vi "Sub Super Duper_12_09_10a_JW.vi"(0 "VISA resource name":refnum<visa-resource-name>="GPIB0::17::INSTR", 1 "Sample Properties:":T7 {"Date Created" format="%<%Y/%m/%d>T"}, 2 "TRF Cluster":T8={"Step 4"=-38.0, "# of Loops"=1.0, "Transfer 2"=FALSE, "Start 4"=-2.0, "Total Points 2"=2, "Start 3"=40.0, "Stop 2"=-40.0, "Step 3"=-1.0, "Loop Step"=0.0, "Integration Time 3"=0, "Loop Wait"=0.0, "First Step"=0.0} {"Loop Wait" format="%<%H:%M:%S>t"; "Integration Time 3" scale=0.0..2.0; "Step 3" format="%.2f"; "Stop 2" format="%.2f"; "Start 3" format="%.2f"; "Start 4" format="%.2f"; "Step 4" format="%.2f"}, 3 "TSP Cluster":T9={"Transport"=FALSE, "Start 2"=0.0, "Stop 3"=-60.0, "Step 2"=-1.0, "Start"=0.0, "Step"=-10.0, "Total Points"=7, "Integration Time"=0} {"Integration Time" scale=0.0..2.0; "Step" format="%.2f"; "Start" format="%.2f"; "Step 2" format="%.2f"; "Stop 3" format="%.2f"; "Start 2" format="%.2f"}, 4 "Compliance Cluster":T4={"Var1 sweep settings"={"sweep spacing (linear: 0)"=0, "sweep mode"=FALSE, "compliance (V)"=100.0, "compliance (A)"=0.001}, "Var1 sweep settings 2"={"sweep spacing (linear: 0)"=0, "sweep mode"=FALSE, "compliance (V)"=100.0, "compliance (A)"=0.001}, "Var2 step settings 2"={"compliance (A)"=0.001, "compliance (V)"=100.0}, "Var2 step settings"={"compliance (A)"=0.001, "compliance (V)"=100.0}} {"Var2 step settings"."compliance (V)" format="%.2f"; "Var2 step settings"."compliance (A)" format="%^.2e"; "Var2 step settings 2"."compliance (V)" format="%.2f"; "Var2 step settings 2"."compliance (A)" format="%^.2e"; "Var1 sweep settings 2"."compliance (A)" format="%^.2e"; "Var1 sweep settings 2"."compliance (V)" format="%.2f"; "Var1 sweep settings 2"."sweep spacing (linear: 0)" items=["linear", "log 10", "log 25", "log 50"]; "Var1 sweep settings"."compliance (A)" format="%^.2e"; "Var1 sweep settings"."compliance (V)" format="%.2f"; "Var1 sweep settings"."sweep spacing (linear: 0)" items=["linear", "log 10", "log 25", "log 50"]}, 5 "error in":errorcluster, 6 "Saved Folder:":path=path "C:/1DATA/2011", 7 "Wait Cluster":T3 {"Wait Time (s)" format="%.1g"; "Wait Countdown" format="%<%H:%M:%S%1u>t"}, 9 "Stop \nCountdown":bool, 11 "Loop Count":dbl, 12 "Gate Current Cluster":T1={"Gate Current (TSP)"={"Y2 axis on/off"=FALSE, "MINIMUM"=0.0, "MAXIMUM"=1.0, "Variable name"="Ig", "LIN or LOG axis"="LIN"}, "Gate Current (TRF)"={"Y2 axis on/off"=FALSE, "MINIMUM"=0.0, "MAXIMUM"=1.0, "Variable name"="Ig", "LIN or LOG axis"="LIN"}} {"Gate Current (TSP)"."MAXIMUM" format="%.9f"; "Gate Current (TSP)"."MINIMUM" format="%.9f"; "Gate Current (TRF)"."MAXIMUM" format="%.9f"; "Gate Current (TRF)"."MINIMUM" format="%.9f"}, 13 "Dielectric Constant":dbl) -> (8 "Status Indicator":bool, 10 "Vt Cluster":T2 {"Id Max" format="%.3g"; "Vt Max" format="%.3g"; "Vt Min" format="%.3g"; "Vt Ratio" format="%.3g"}, 14 "VISA resource name out":refnum<visa-resource-name>, 15 "TRF Path":path, 16 "TSP Path":path, 17 "Graph Cluster":T5, 18 "Char Cluster":T6 {"Mobility-Lin" format="%#_4e"; "On/Off" format="%#_4e"; "Mobility-Sat" format="%#_4e"}, 19 "error out":errorcluster)   [LabVIEW 2012]
uses:
  <vilib>/Platform/TimedLoop/XDataNode/wakeup.ctl
  <vilib>/Platform/TimedLoop/XDataNode/XDNodeRunTimeDep.lvlib
  <vilib>/Platform/TimedLoop/XDataNode/nitl_modes.ctl
  <vilib>/Platform/TimedLoop/XDataNode/timing_clust.ctl
  <vilib>/Platform/TimedLoop/XDataNode/XDataNode.xnode
panel:
  out "LKG Path":path
  # "Vg Sweep"
  # "Vd Step"
  # "Loops and Integration Time"
  # "Device Characteristics"
  # "Sample Properties:"
  # "%"
  # "nm"
  # "Device Properties:"
  # "um"
  # "um"
  # "Vg Step"
  # "Vd Step"
  # "Integration Time"
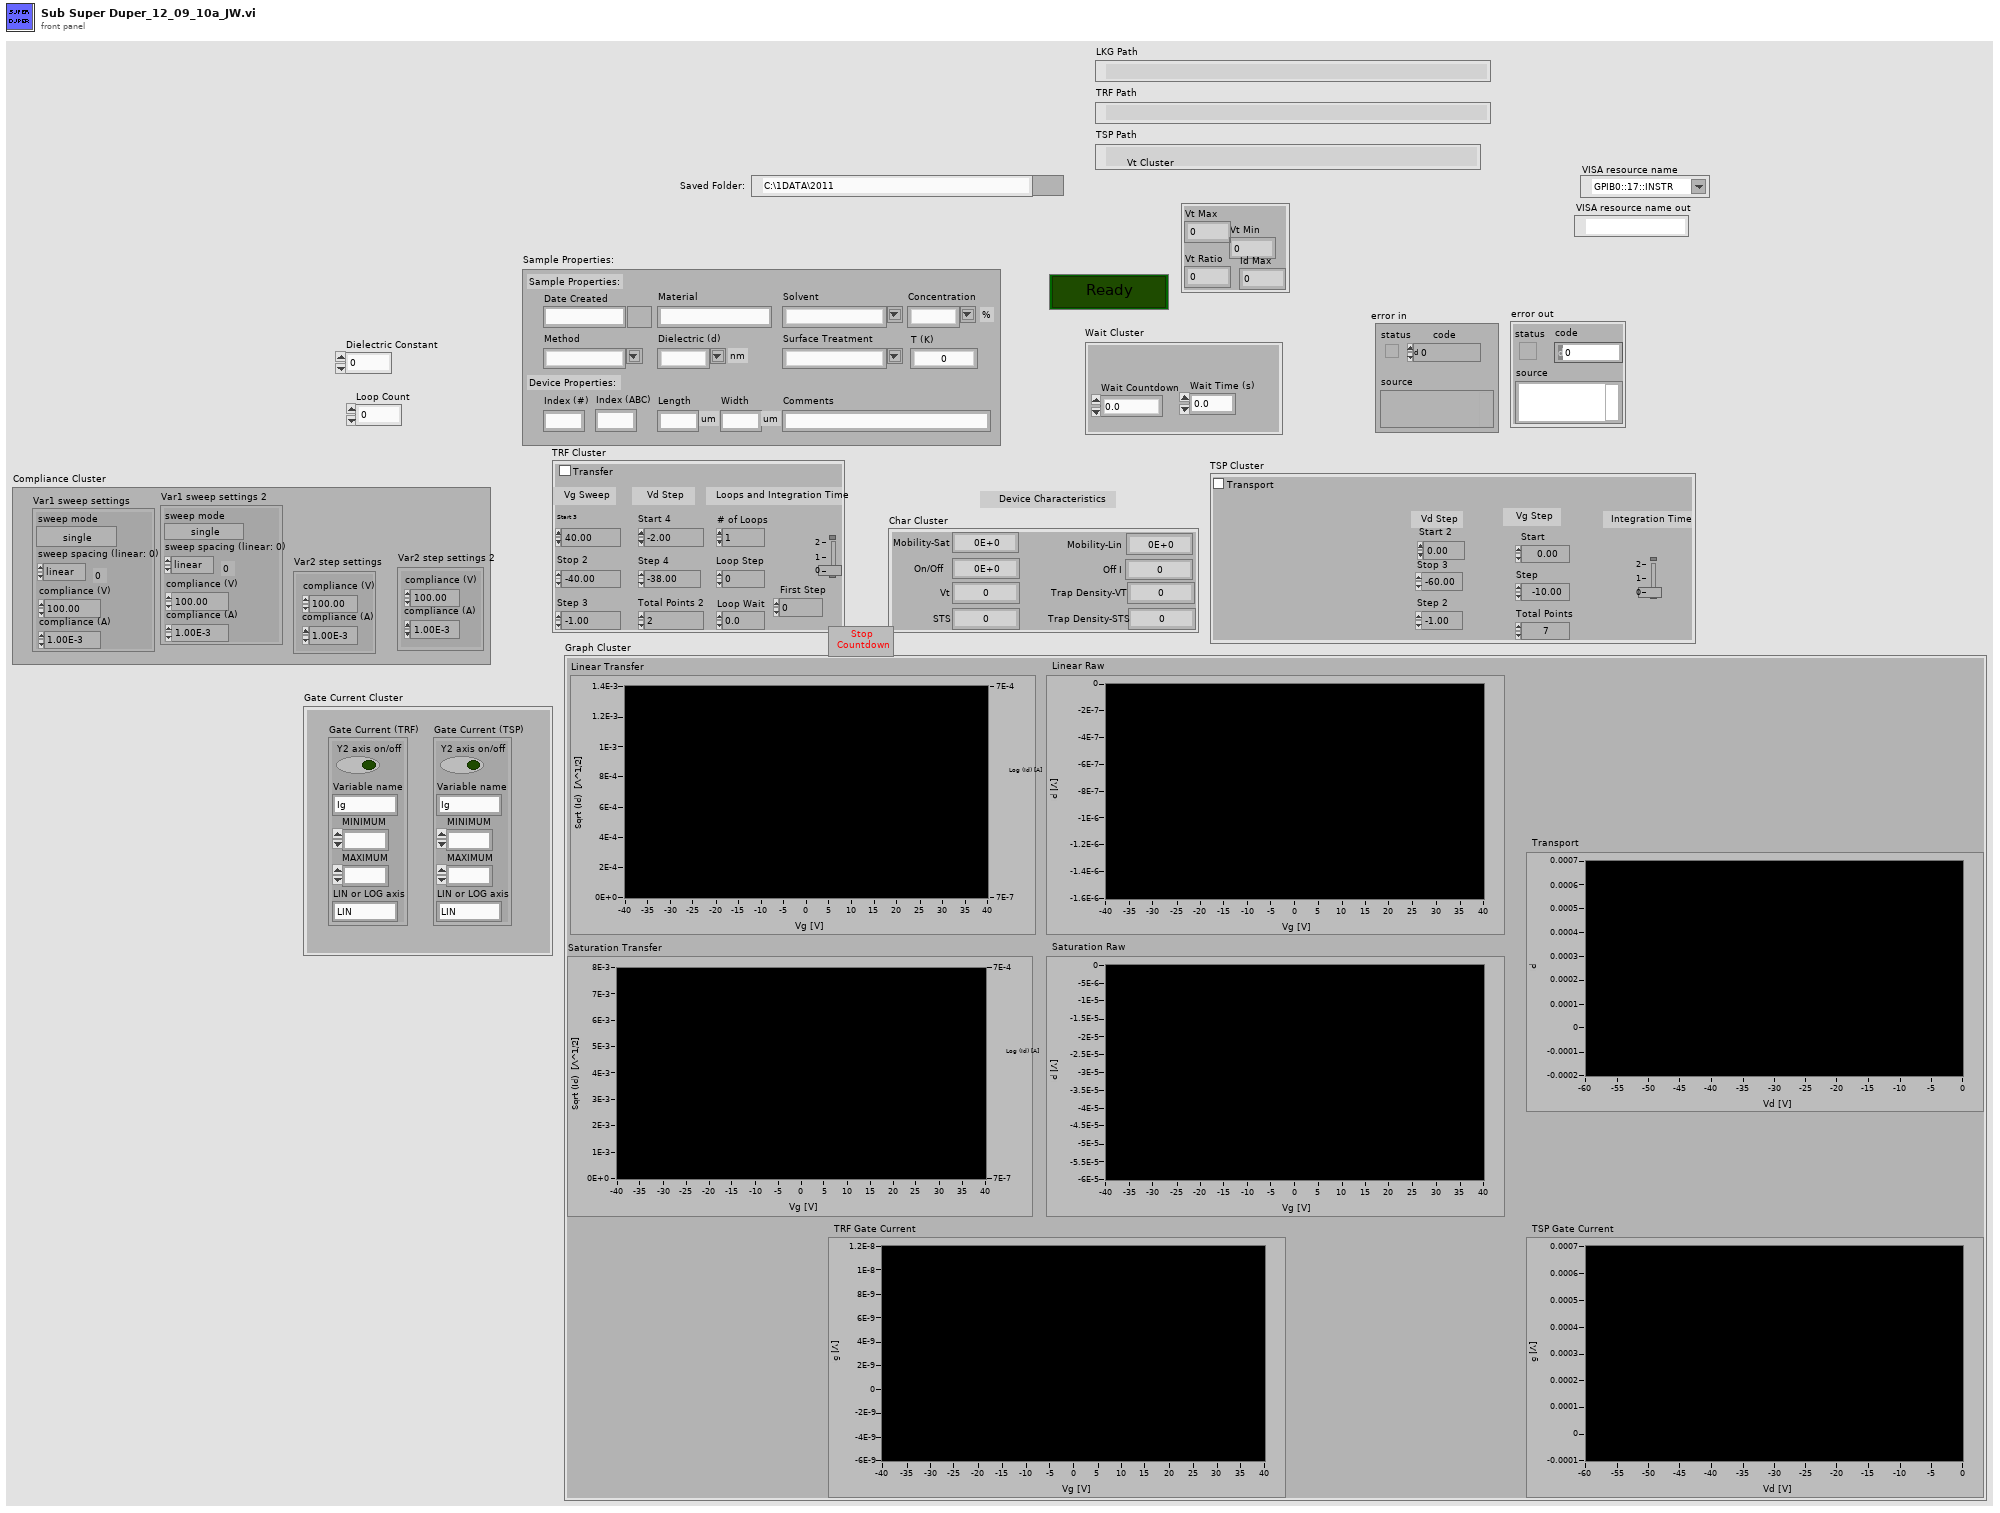
[diagram p1: front panel]
types:
  T1 = cluster{"Gate Current (TSP)":cluster{"Y2 axis on/off":bool, "MINIMUM":ext, "MAXIMUM":ext, "Variable name":string, "LIN or LOG axis":string}, "Gate Current (TRF)":cluster{"Y2 axis on/off":bool, "MINIMUM":ext, "MAXIMUM":ext, "Variable name":string, "LIN or LOG axis":string}}
  T2 = cluster{"Vt Max":i32, "Vt Min":i32, "Vt Ratio":i32, "Id Max":i32}
  T3 = cluster{"Wait Countdown":dbl, "Wait Time (s)":dbl}
  T4 = cluster{"Var1 sweep settings":cluster{"sweep spacing (linear: 0)":u16, "sweep mode":bool, "compliance (V)":dbl, "compliance (A)":dbl}, "Var1 sweep settings 2":cluster{"sweep spacing (linear: 0)":u16, "sweep mode":bool, "compliance (V)":dbl, "compliance (A)":dbl}, "Var2 step settings 2":cluster{"compliance (A)":dbl, "compliance (V)":dbl}, "Var2 step settings":cluster{"compliance (A)":dbl, "compliance (V)":dbl}}
  T5 = cluster{"Linear Transfer":cluster{dbl[], "trace":dbl[]}[], "Linear Raw":cluster{dbl[], dbl[]}[], "Saturation Transfer":cluster{dbl[], "trace":dbl[]}[], "Saturation Raw":cluster{dbl[], dbl[]}[], "Transport":cluster{dbl[], dbl[]}[], "TRF Gate Current":cluster{dbl[], dbl[]}[], "TSP Gate Current":cluster{dbl[], dbl[]}[]}
  T6 = cluster{"Mobility-Sat":dbl, "Mobility-Lin":dbl, "On/Off ":dbl, "Off I":dbl, "Vt":dbl, "STS":dbl, "Trap Density-VT":dbl, "Trap Density-STS":dbl}
  T7 = cluster{"Date Created":timestamp, "Material":string, "Solvent":string, "Concentration":string, "Method":string, "Dielectric (d)":string, "Index (#)":string, "Index (ABC)":string, "Length":string, "Width":string, "Surface Treatment":string, "Comments":string, "T (K)":dbl}
  T8 = cluster{"Step 4":dbl, "# of Loops":dbl, "Transfer 2":bool, "Start 4":dbl, "Total Points 2":u16, "Start 3":dbl, "Stop 2":dbl, "Step 3":dbl, "Loop Step":dbl, "Integration Time 3":u32, "Loop Wait":dbl, "First Step":dbl}
  T9 = cluster{"Transport":bool, "Start 2":dbl, "Stop 3":dbl, "Step 2":dbl, "Start":dbl, "Step":dbl, "Total Points":u16, "Integration Time":u32}
  T10 = typedef "XDNodeRunTimeDep.lvlib/timing_clust.ctl" = cluster{"Expected End [f-1]":u64, "Actual End [f-1]":u64, "Finished Late? [f-1]":bool, "Expected End [i-1]":u64, "Actual End [i-1]":u64, "Finished Late? [i-1]":bool, "Expected Start [i]":u64, "Actual Start [i]":u64, "Expected Start [f]":u64, "Actual Start [f]":u64, "Source Name":string, "Structure Name":string, "Period":i64, "Deadline":i64, "Offset":i64, "Start":i64, "Priority":i32, "Timeout":i32, "Mode":T11, "Wakeup Reason":T12, "Error":errorcluster, "Source Type":string, "Secondary Source Type":string, "Global End Time":u64, "Global Start Time":u64, "Frame Duration":u64, "Iteration Duration":u64, "Assigned CPU":i32, "I/O Scan Engine Mode":u32}
  T11 = typedef "XDNodeRunTimeDep.lvlib/nitl_modes.ctl" = enum32{"No Change", "Process missed periods, maintain original phase", "Discard missed periods, maintain original phase", "Process missed periods, ignore original phase", "Discard missed periods, ignore original phase"}
  T12 = typedef "XDNodeRunTimeDep.lvlib/wakeup.ctl" = enum32{"Normal", "Aborted", "Asynchronous wakeup", "Timing source error", "Timed loop error", "Timeout"}
  T13 = cluster{"sweep spacing (linear: 0)":u16, "sweep mode":bool, "compliance (V)":dbl, "compliance (A)":dbl}
  T14 = cluster{"compliance (A)":dbl, "compliance (V)":dbl}
  T15 = cluster{"Y2 axis on/off":bool, "MINIMUM":ext, "MAXIMUM":ext, "Variable name":string, "LIN or LOG axis":string}
  T16 = cluster{"Start 3":dbl, "Stop 2":dbl, "Step 3":dbl, "sweep spacing (linear: 0)":u16, "sweep mode":bool, "compliance (V)":dbl, "compliance (A)":dbl}
  T17 = cluster{"compliance (A)":dbl, "compliance (V)":dbl, "Start 4":dbl, "Total Points 2":u16, dbl}
  T18 = cluster{"Vt Max":i32, "Vt Min":i32, "Vt Ratio":i32, "Id Max":dbl}
  T19 = cluster{"Mobility-Sat":dbl, "Mobility-Lin":dbl, "On/Off Current":dbl, "Off I":dbl, "Vt":dbl, "STS":dbl, "Trap Density-VT":dbl, "Trap Density-STS":dbl}
  T20 = cluster{"Linear Sqrt":cluster{dbl[], "trace":dbl[]}[], "Linear Log":cluster{dbl[], "trace":dbl[]}[], "Linear Raw":cluster{dbl[], dbl[]}[], "Saturation Sqrt":cluster{dbl[], "trace":dbl[]}[], "Saturation Log":cluster{dbl[], "trace":dbl[]}[], "Saturation Raw":cluster{dbl[], "trace":dbl[]}[], "Gate Current":cluster{dbl[], "trace":dbl[]}[]}
  T21 = cluster{"Start 2":dbl, "Stop 3":dbl, "Step 2":dbl, "sweep spacing (linear: 0)":u16, "sweep mode":bool, "compliance (V)":dbl, "compliance (A)":dbl}
  T22 = cluster{"compliance (A)":dbl, "compliance (V)":dbl, "Start":dbl, "Total Points":u16, "Step":dbl}
  T23 = cluster{"Transport":cluster{dbl[], dbl[]}[], "Gate Current":cluster{dbl[], dbl[]}[]}
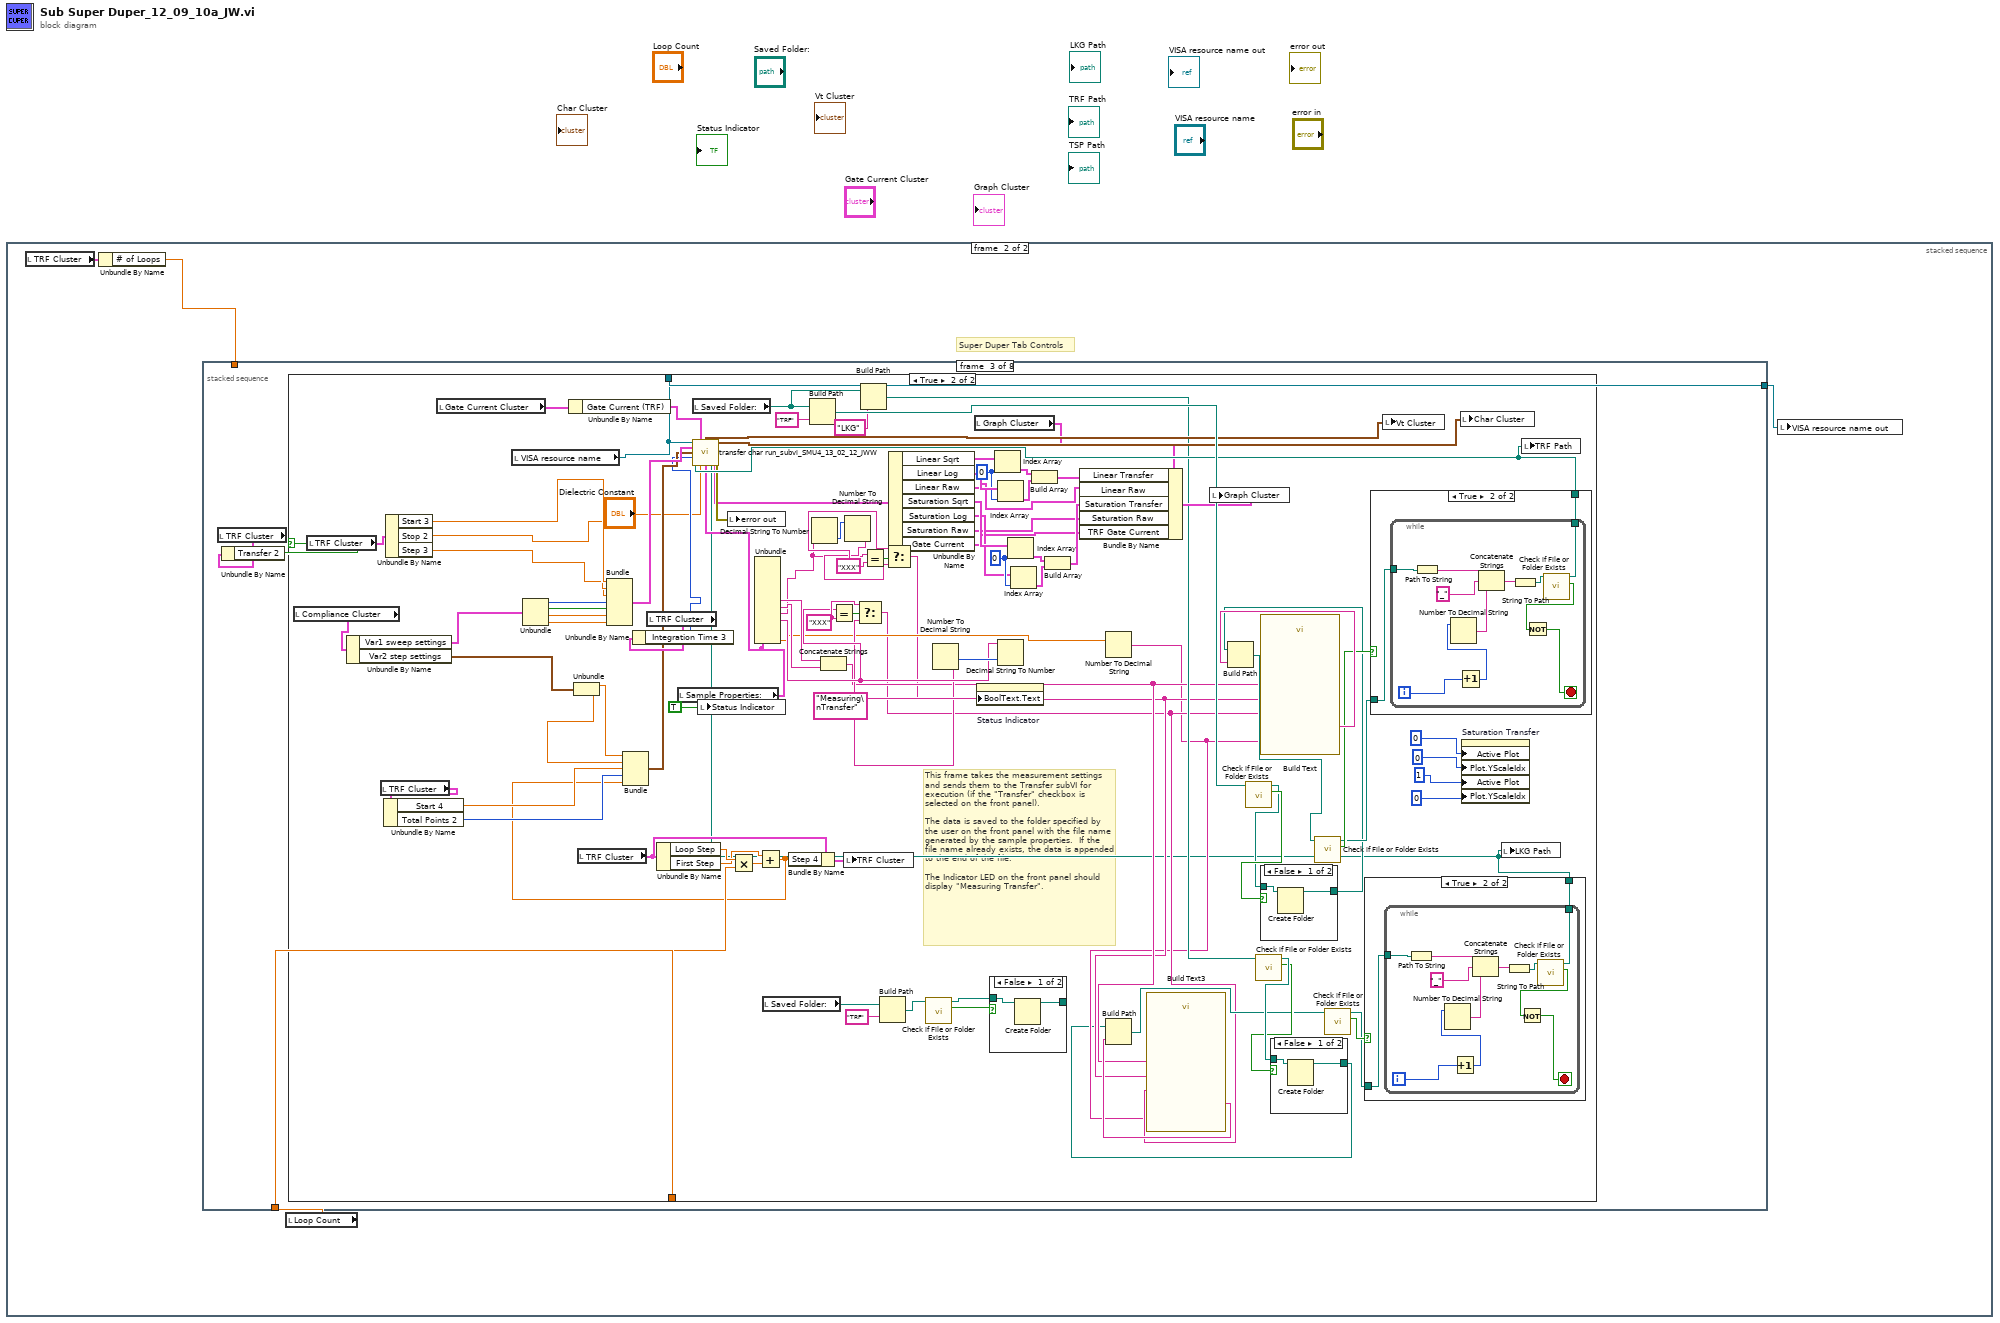
[diagram p0: block diagram]
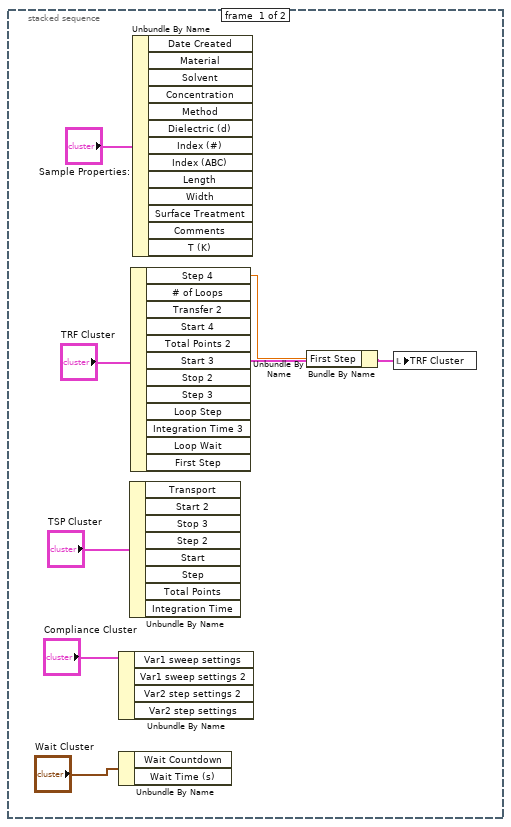
[diagram p2: hidden frame]
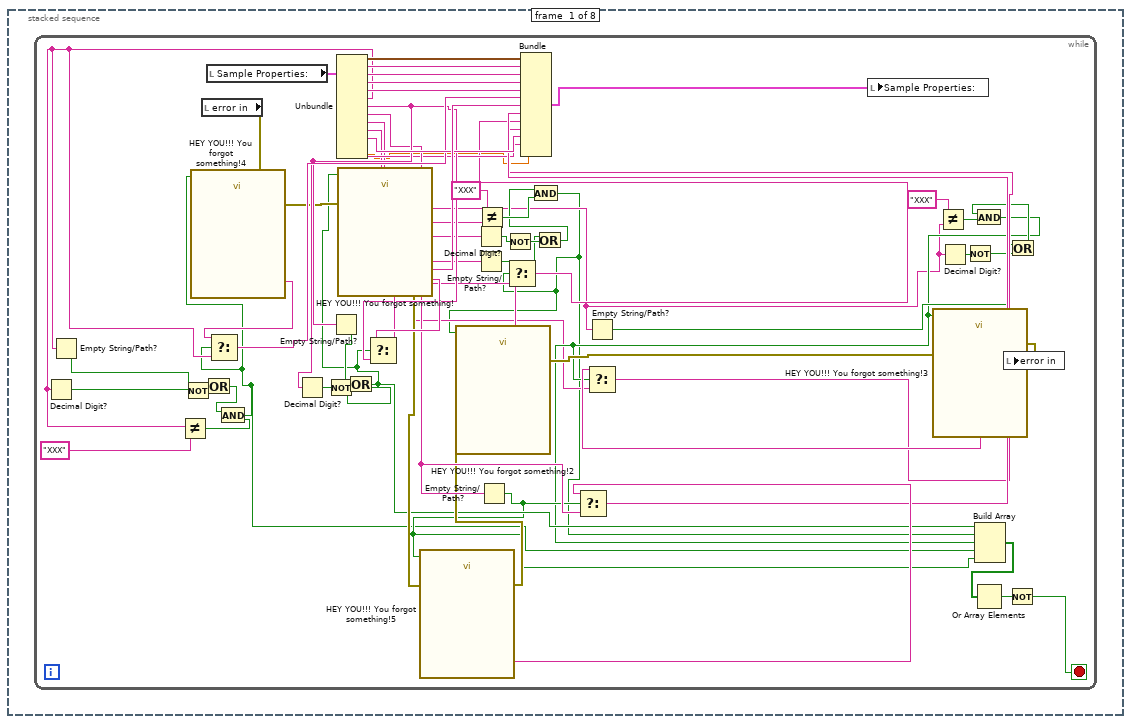
[diagram p3: hidden frame]
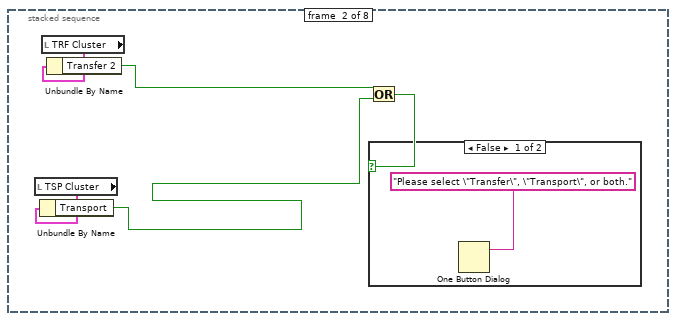
[diagram p4: hidden frame]
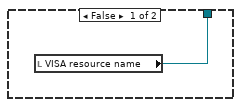
[diagram p6: hidden frame]
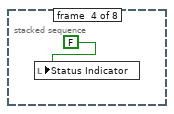
[diagram p12: hidden frame]
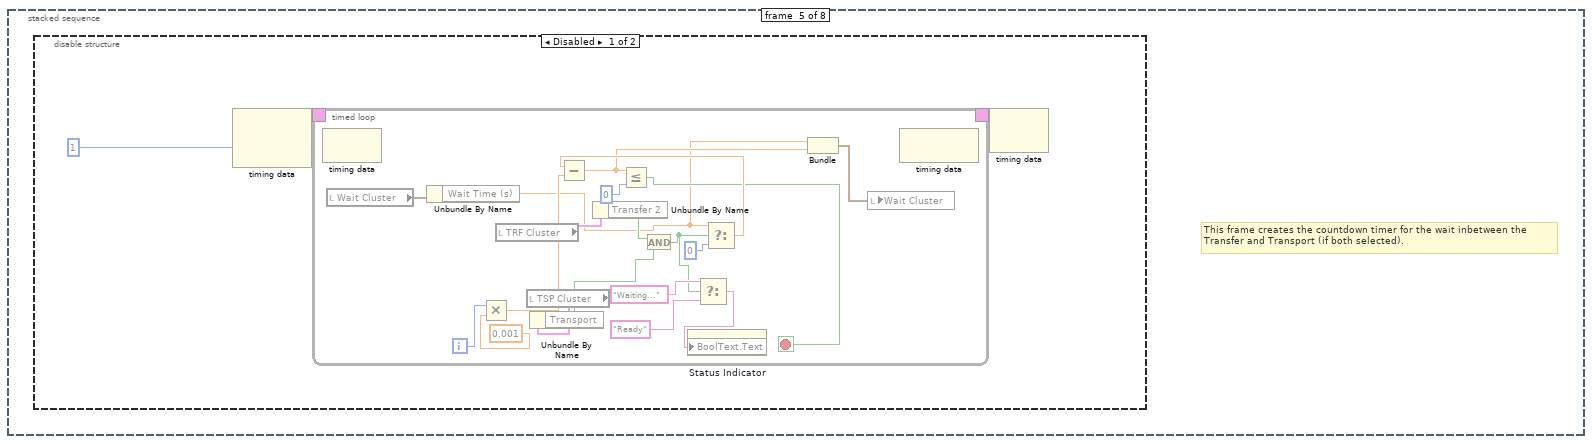
[diagram p13: hidden frame]
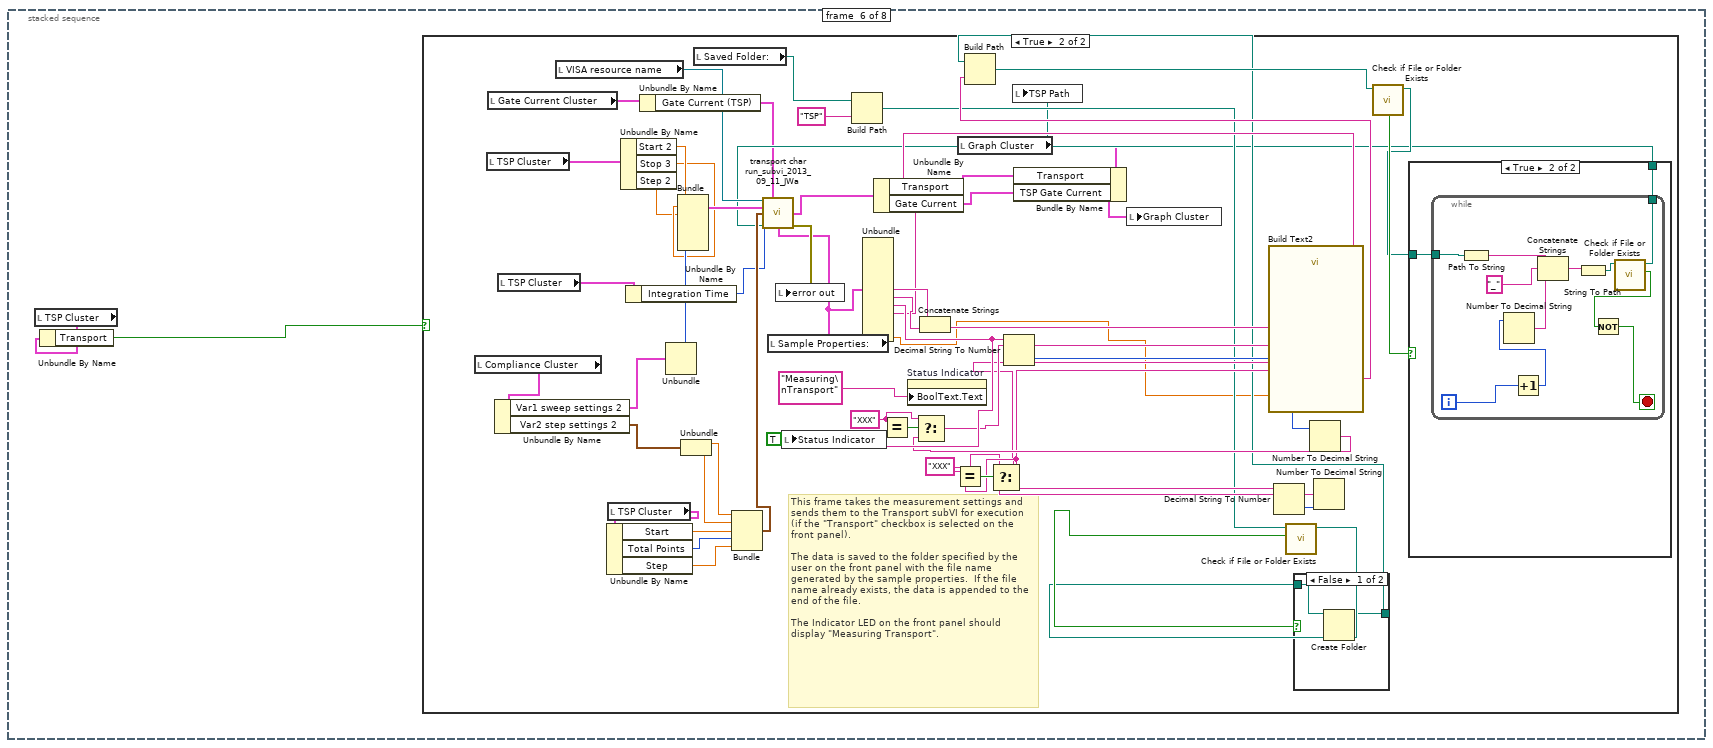
[diagram p15: hidden frame]
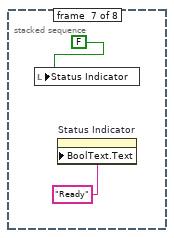
[diagram p19: hidden frame]
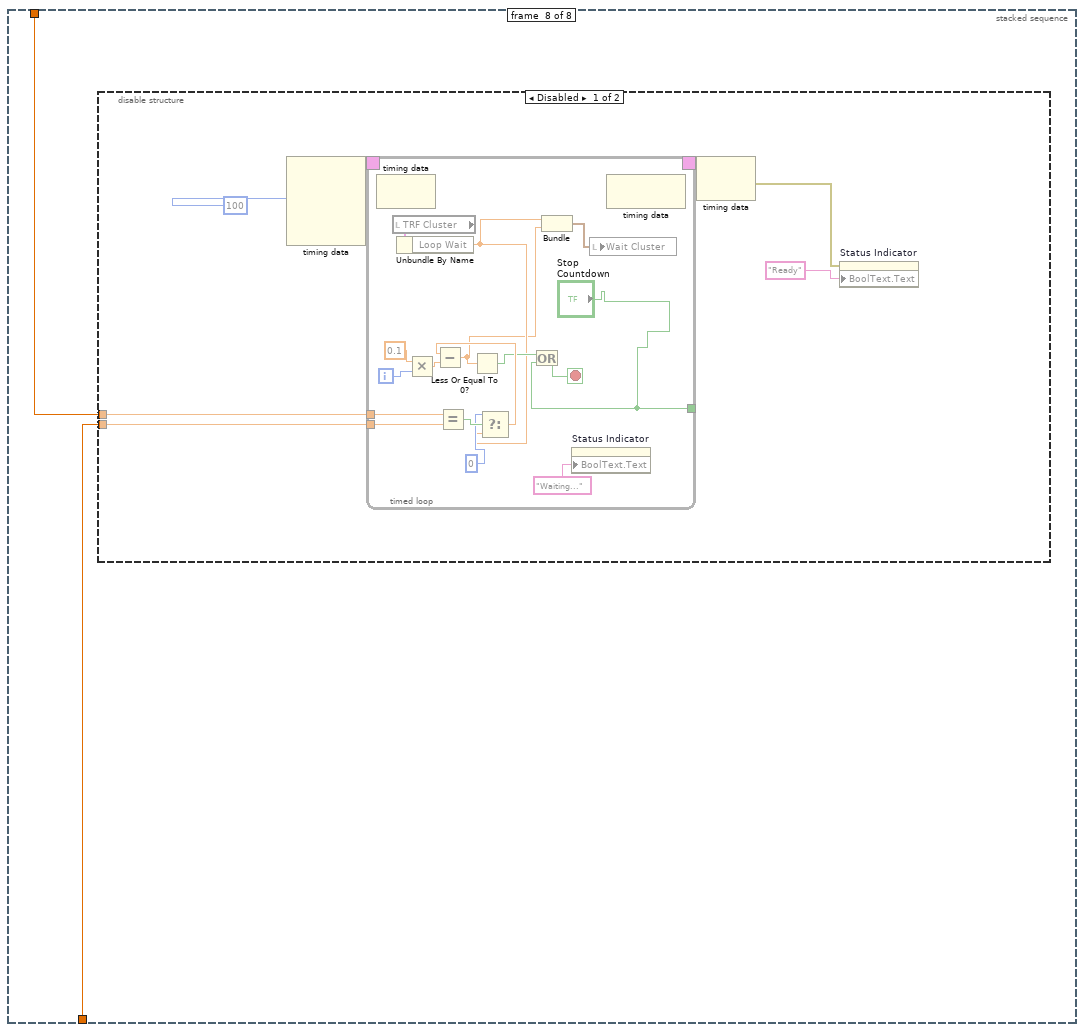
[diagram p20: hidden frame]
diagram:
  n1 = stacked-sequence {
    frame #0 {
      n2 = Unbundle By Name("Compliance Cluster") -> ()  [unwired: 4 out]
      n3 = Unbundle By Name("Wait Cluster") -> ()  [unwired: 2 out]
      n4 = Unbundle By Name("TSP Cluster") -> ()  [unwired: 8 out]
      n5 = Unbundle By Name("TRF Cluster") -> ("Step 4"=w7:dbl)  [unwired: 11 out]
      n6 = Unbundle By Name("Sample Properties:") -> ()  [unwired: 13 out]
      n7 = Bundle By Name(cluster="TRF Cluster", "First Step"=w7) -> (w5:T8)
      n8 = local write "TRF Cluster"(w5) -> ()
    }
    frame #1 {
      # "Super Duper Tab Controls"
      n9 = local read "TRF Cluster"() -> (w11:T8)
      n10 = Unbundle By Name(w11) -> ("# of Loops"=w10:dbl)
      n11 = local read "Loop Count"() -> (w8:dbl)
      n12 = stacked-sequence {
        tunnel: w8 -> [_ _ w81 _ _ _ _ w333]
        tunnel: w10 -> [_ _ _ _ _ _ _ w332]
        tunnel: [_ _ w78 _ _ _ _ _] -> w9
        frame #0 {
          n13 = while {
            stop <- w37 stop-if-true
            n14 = local read "error in"() -> (w43:errorcluster)
            n15 = local read "Sample Properties:"() -> (w66:T7)
            n16 = Unbundle(w66) -> ("Date Created"=w67:timestamp, "Material"=w68:string, "Solvent"=w69:string, "Concentration"=w70:string, "Method"=w71:string, "Dielectric (d)"=w26:string, "Index (#)"=w56:string, "Index (ABC)"=w53:string, "Length"=w21:string, "Width"=w14:string, "Surface Treatment"=w59:string, "Comments"=w51:string, "T (K)"=w12:dbl)
            n17 = Decimal Digit?(1:w26) -> (0:w34:bool)
            n18 = Empty String/Path?(string/path=w26) -> (empty?=w28:bool)
            n19 = Not Equal?(x=w26, y="XXX") -> (x != y?=w25:bool)
            n20 = Not(x=w34) -> (.not. x?=w31:bool)
            n21 = Or(x=w28, y=w31) -> (x .or. y?=w24:bool)
            n22 = And(x=w24, y=w25) -> (x .and. y?=w23:bool)
            n23 = call "HEY YOU!!! You forgot something!4"("Enable"=w23, "error in (no error)"=w43) -> ("Dielectric (d)"=w58:string, "error out"=w42:errorcluster)  [unwired: 15 in, 1 out]
            n24 = Select(t=w58, s=w23, f=w26) -> (s? t:f=w57:string)
            n25 = Decimal Digit?(1:w56) -> (0:w47:bool)
            n26 = Not(x=w47) -> (.not. x?=w46:bool)
            n27 = Empty String/Path?(string/path=w56) -> (empty?=w55:bool)
            n28 = Or(x=w55, y=w46) -> (x .or. y?=w41:bool)
            n29 = call "HEY YOU!!! You forgot something!"("Enable"=w41, "error in (no error)"=w42) -> ("Index (#)"=w65:string, "error out"=w45:errorcluster)  [unwired: 15 in, 1 out]
            n30 = Select(t=w65, s=w41, f=w56) -> (s? t:f=w62:string)
            n31 = Decimal Digit?(1:w21) -> (0:w36:bool)
            n32 = Empty String/Path?(string/path=w21) -> (empty?=w30:bool)
            n33 = Not Equal?(x="XXX", y=w21) -> (x != y?=w20:bool)
            n34 = Empty String/Path?(string/path=w53) -> (empty?=w40:bool)
            n35 = call "HEY YOU!!! You forgot something!5"("Enable"=w40, "error in (no error)"=w45) -> ("Index (ABC)"=w54:string, "error out"=w44:errorcluster)  [unwired: 15 in, 1 out]
            n36 = Not(x=w36) -> (.not. x?=w33:bool)
            n37 = Or(x=w30, y=w33) -> (x .or. y?=w19:bool)
            n38 = And(x=w19, y=w20) -> (x .and. y?=w13:bool)
            n39 = call "HEY YOU!!! You forgot something!2"("Enable"=w13, "error in (no error)"=w44) -> ("Length"=w64:string, "error out"=w61:errorcluster)  [unwired: 15 in, 1 out]
            n40 = Select(t=w64, s=w13, f=w21) -> (s? t:f=w50:string)
            n41 = Select(t=w54, s=w40, f=w53) -> (s? t:f=w52:string)
            n42 = Empty String/Path?(string/path=w14) -> (empty?=w29:bool)
            n43 = Not Equal?(x="XXX", y=w14) -> (x != y?=w18:bool)
            n44 = Decimal Digit?(1:w14) -> (0:w35:bool)
            n45 = Not(x=w35) -> (.not. x?=w32:bool)
            n46 = Or(x=w29, y=w32) -> (x .or. y?=w17:bool)
            n47 = And(x=w17, y=w18) -> (x .and. y?=w16:bool)
            n48 = call "HEY YOU!!! You forgot something!3"("Enable"=w16, "error in (no error)"=w61) -> ("Width"=w63:string, "error out"=w60:errorcluster)  [unwired: 15 in, 1 out]
            n49 = Select(t=w63, s=w16, f=w14) -> (s? t:f=w49:string)
            n50 = Bundle("Date Created"=w67, "Material"=w68, "Solvent"=w69, "Concentration"=w70, "Method"=w71, "Dielectric (d)"=w57, "Index (#)"=w62, "Index (ABC)"=w52, "Length"=w50, "Width"=w49, "Surface Treatment"=w59, "Comments"=w51, "T (K)"=w12) -> (w48:T7)  [unwired: 1 in]
            n51 = local write "Sample Properties:"(w48) -> ()
            n52 = Build Array(w41, w13, w16, w23, w40) -> (w39:bool[])
            n53 = Or Array Elements(Boolean array=w39) -> (logical OR=w38:bool)
            n54 = local write "error in"(w60) -> ()
            n55 = Not(x=w38) -> (.not. x?=w37:bool)
          }
        }
        frame #1 {
          n56 = local read "TSP Cluster"() -> (w73:T9)
          n57 = Unbundle By Name(w73) -> ("Transport"=w72:bool)
          n58 = local read "TRF Cluster"() -> (w75:T8)
          n59 = Unbundle By Name(w75) -> ("Transfer 2"=w74:bool)
          n60 = Or(x=w74, y=w72) -> (x .or. y?=w76:bool)
          n61 = case shown="False" w76 {
            frame False {
              n62 = One Button Dialog(message="Please select \"Transfer\", \"Transport\", or both.") -> ()  [unwired: 1 in, 1 out]
            }
            frame True {
            }
          }
        }
        frame #2 {
          n63 = local read "TRF Cluster"() -> (w79:T8)
          n64 = Unbundle By Name(w79) -> ("Transfer 2"=w80:bool)
          n65 = case shown="True" w80 {
            tunnel: w81 -> [_ w138]
            tunnel: [w82 w132] -> w78
            frame False {
              n66 = local read "VISA resource name"() -> (w82:refnum<visa-resource-name>)
            }
            frame True {
              w113 = 0
              w119 = 0
              w164 = "XXX"
              w167 = "XXX"
              # "This frame takes the measurement settings and sends them to the Transfer subVI for execution (if the \"Transfer\" checkbox is selected on the front panel).\n\nThe data is saved to the folder specified by the user on the front panel with the file name generated by the sample properties.  If the file name already exists, the data is appended to the end of the file.\n\nThe Indicator LED on the front panel should display \"Measuring Transfer\"."
              n67 = local read "Compliance Cluster"() -> (w143:T4)
              n68 = local read "TRF Cluster"() -> (w148:T8)
              n69 = Unbundle By Name(w143) -> ("Var1 sweep settings"=w141:T13, "Var2 step settings"=w142:T14)
              n70 = local read "TRF Cluster"() -> (w151:T8)
              n71 = Unbundle By Name(w151) -> ("Start 4"=w150:dbl, "Total Points 2"=w149:u16)
              n72 = Unbundle By Name(w148) -> ("Start 3"=w147:dbl, "Stop 2"=w146:dbl, "Step 3"=w145:dbl)
              n73 = local read "Gate Current Cluster"() -> (w84:T1)
              n74 = local read "VISA resource name"() -> (w132:refnum<visa-resource-name>)
              n75 = Unbundle(w141) -> ("sweep spacing (linear: 0)"=w184:u16, "sweep mode"=w183:bool, "compliance (V)"=w182:dbl, "compliance (A)"=w181:dbl)
              n76 = Unbundle By Name(w84) -> ("Gate Current (TRF)"=w83:T15)
              n77 = Unbundle(w142) -> ("compliance (A)"=w180:dbl, "compliance (V)"=w179:dbl)
              n78 = local read "TRF Cluster"() -> (w133:T8)
              n79 = Bundle("Start 3"=w147, "Stop 2"=w146, "Step 3"=w145, "sweep spacing (linear: 0)"=w184, "sweep mode"=w183, "compliance (V)"=w182, "compliance (A)"=w181) -> (w131:T16)  [unwired: 1 in]
              n80 = local read "TRF Cluster"() -> (w144:T8)
              n81 = Unbundle By Name(w144) -> ("Integration Time 3"=w129:u32)
              n82 = Unbundle By Name(w133) -> ("Loop Step"=w136:dbl, "First Step"=w135:dbl)
              n83 = local read "Sample Properties:"() -> (w127:T7)
              n84 = local read "Saved Folder:"() -> (w99:path)
              n85 = local write "Status Indicator"(TRUE) -> ()
              n86 = Multiply(x=w136, y=w138) -> (x*y=w139:dbl)
              n87 = Unbundle(w127) -> ("Index (#)"=w175:string, "Index (ABC)"=w174:string, "Length"=w161:string, "Width"=w163:string, "T (K)"=w140:dbl)  [unwired: 8 out]
              n88 = Add(x=w135, y=w139) -> (x+y=w134:dbl)
              n89 = Bundle("compliance (A)"=w180, "compliance (V)"=w179, "Start 4"=w150, "Total Points 2"=w149, w134) -> (w130:T17)  [unwired: 1 in]
              n90 = local read "Saved Folder:"() -> (w106:path)
              n91 = Bundle By Name(cluster=w133, "Step 4"=w134) -> (w137:T8)
              n92 = Build Path(base path=w99, name or relative path="TRF") -> (appended path=w157:path)
              n93 = Decimal String To Number(string=w161) -> (number=w170:i32)  [unwired: 2 in, 1 out]
              n94 = Concatenate Strings(w175, w174) -> (w90:string)
              n95 = Equal?(x=w163, y=w164) -> (x = y?=w165:bool)
              n96 = local write "TRF Cluster"(w137) -> ()
              n97 = Number To Decimal String(number=w170) -> (decimal integer string=w166:string)  [unwired: 1 in]
              n98 = Build Path(base path=w99, name or relative path="LKG") -> (appended path=w95:path)
              n99 = Equal?(x=w161, y=w167) -> (x = y?=w168:bool)
              n100 = Build Path(base path=w106, name or relative path="TRF") -> (appended path=w104:path)
              n101 = Select(t=w167, s=w168, f=w166) -> (s? t:f=w89:string)
              n102 = call <vilib>:"Check if File or Folder Exists.vi"("path"=w104) -> ("file or folder exists?"=w102:bool, "dup path"=w103:path)  [unwired: 8 in, 1 out]
              n103 = local read "Graph Cluster"() -> (w122:T5)
              n104 = property on="Status Indicator" class="Bool (strict)"("BoolText.Text"="Measuring\nTransfer") -> ()  [unwired: 2 in, 2 out]
              n105 = case shown="False" w102 {
                tunnel: w103 -> [w203 w204]
                tunnel: [w202 w204] -> _
                frame False {
                  n106 = Create Folder(path (use dialog)=w203) -> (created path=w202:path)  [unwired: 2 in, 2 out]
                }
                frame True {
                }
              }
              n107 = Decimal String To Number(string=w163) -> (number=w169:i32)  [unwired: 2 in, 1 out]
              n108 = Number To Decimal String(number=w169) -> (decimal integer string=w162:string)  [unwired: 1 in]
              n109 = Select(t=w164, s=w165, f=w162) -> (s? t:f=w88:string)
              n110 = Number To Decimal String(number=w140) -> (decimal integer string=w87:string)  [unwired: 1 in]
              n111 = call "Build Text3"("T"=w87, "Index"=w90, "Length"=w89, "Width"=w88) -> ("Result"=w91:string)  [unwired: 10 in, 1 out]
              n112 = call <vilib>:"Check if File or Folder Exists.vi"("path"=w157) -> ("file or folder exists?"=w159:bool, "dup path"=w158:path)  [unwired: 8 in, 1 out]
              n113 = call <vilib>:"Check if File or Folder Exists.vi"("path"=w95) -> ("file or folder exists?"=w96:bool, "dup path"=w97:path)  [unwired: 8 in, 1 out]
              n114 = call "Build Text"("T"=w87, "Index"=w90, "Length"=w89, "Width"=w88) -> ("Result"=w178:string)  [unwired: 10 in, 1 out]
              n115 = case shown="False" w159 {
                tunnel: w158 -> [w206 w207]
                tunnel: [w205 w207] -> w156
                frame False {
                  n116 = Create Folder(path (use dialog)=w206) -> (created path=w205:path)  [unwired: 2 in, 2 out]
                }
                frame True {
                }
              }
              n117 = Build Path(base path=w156, name or relative path=w178) -> (appended path=w172:path)
              n118 = case shown="False" w96 {
                tunnel: w97 -> [w200 w201]
                tunnel: [w199 w201] -> w86
                frame False {
                  n119 = Create Folder(path (use dialog)=w200) -> (created path=w199:path)  [unwired: 2 in, 2 out]
                }
                frame True {
                }
              }
              n120 = Build Path(base path=w86, name or relative path=w91) -> (appended path=w94:path)
              n121 = call <vilib>:"Check if File or Folder Exists.vi"("path"=w172) -> ("file or folder exists?"=w173:bool, "dup path"=w171:path)  [unwired: 8 in, 1 out]
              n122 = call <vilib>:"Check if File or Folder Exists.vi"("path"=w94) -> ("file or folder exists?"=w93:bool, "dup path"=w92:path)  [unwired: 8 in, 1 out]
              n123 = case shown="True" w93 {
                tunnel: w92 -> [w185 w187]
                tunnel: [w185 w186] -> w85
                frame False {
                }
                frame True {
                  n124 = while {
                    tunnel: w187 -> [w189]
                    tunnel: [w188] -> w186
                    i -> [w191]
                    stop <- w192 stop-if-true
                    n125 = Path To String(path=w189) -> (string=w198:string)
                    n126 = Increment(x=w191) -> (x+1=w190:i32)
                    n127 = Number To Decimal String(number=w190) -> (decimal integer string=w196:string)  [unwired: 1 in]
                    n128 = Concatenate Strings(w198, "_", w196) -> (w195:string)
                    n129 = String To Path(string=w195) -> (path=w194:path)
                    n130 = call <vilib>:"Check if File or Folder Exists.vi"("path"=w194) -> ("file or folder exists?"=w193:bool, "dup path"=w188:path)  [unwired: 8 in, 1 out]
                    n131 = Not(x=w193) -> (.not. x?=w192:bool)
                  }
                }
              }
              n132 = case shown="True" w173 {
                tunnel: w171 -> [w208 w210]
                tunnel: [w208 w209] -> w128
                frame False {
                }
                frame True {
                  n133 = while {
                    tunnel: w210 -> [w212]
                    tunnel: [w211] -> w209
                    i -> [w214]
                    stop <- w215 stop-if-true
                    n134 = Path To String(path=w212) -> (string=w221:string)
                    n135 = Increment(x=w214) -> (x+1=w213:i32)
                    n136 = Number To Decimal String(number=w213) -> (decimal integer string=w219:string)  [unwired: 1 in]
                    n137 = Concatenate Strings(w221, "_", w219) -> (w218:string)
                    n138 = String To Path(string=w218) -> (path=w217:path)
                    n139 = call <vilib>:"Check if File or Folder Exists.vi"("path"=w217) -> ("file or folder exists?"=w216:bool, "dup path"=w211:path)  [unwired: 8 in, 1 out]
                    n140 = Not(x=w216) -> (.not. x?=w215:bool)
                  }
                }
              }
              n141 = call "transfer char run_subvi_SMU4_13_02_12_JWW.vi"("VISA session"=w132, "Y2 axis settings"=w83, "LKG Path"=w85, "Var1 sweep settings"=w131, "Var2 step settings"=w130, "integration time"=w129, "Input Path"=w128, "Dielectric Constant"="Dielectric Constant", "Sample Properties:"=w127) -> ("Check Cluster"=w124:T18, "Output"=w125:T19, "Graph Cluster"=w123:T20, "error?"=w126:errorcluster)  [unwired: 3 in]
              n142 = local write "error out"(w126) -> ()
              n143 = Unbundle By Name(w123) -> ("Linear Sqrt"=w121:cluster{dbl[], "trace":dbl[]}[], "Linear Log"=w120:cluster{dbl[], "trace":dbl[]}[], "Linear Raw"=w109:cluster{dbl[], dbl[]}[], "Saturation Sqrt"=w112:cluster{dbl[], "trace":dbl[]}[], "Saturation Log"=w111:cluster{dbl[], "trace":dbl[]}[], "Saturation Raw"=w108:cluster{dbl[], "trace":dbl[]}[], "Gate Current"=w100:cluster{dbl[], "trace":dbl[]}[])
              n144 = Index Array(array=w121, index=w119) -> (element=w118:cluster{dbl[], "trace":dbl[]})
              n145 = Index Array(array=w120, index=w119) -> (element=w117:cluster{dbl[], "trace":dbl[]})
              n146 = Index Array(array=w112, index=w113) -> (element=w114:cluster{dbl[], "trace":dbl[]})
              n147 = Index Array(array=w111, index=w113) -> (element=w115:cluster{dbl[], "trace":dbl[]})
              n148 = Build Array(w118, w117) -> (w116:cluster{dbl[], "trace":dbl[]}[])
              n149 = Build Array(w114, w115) -> (w110:cluster{dbl[], "trace":dbl[]}[])
              n150 = Bundle By Name(cluster=w122, "Linear Transfer"=w116, "Linear Raw"=w109, "Saturation Transfer"=w110, "Saturation Raw"=w108, "TRF Gate Current"=w100) -> (w107:T5)
              n151 = local write "Graph Cluster"(w107) -> ()
              n152 = local write "Vt Cluster"(w124) -> ()
              n153 = local write "Char Cluster"(w125) -> ()
              n154 = property on="Saturation Transfer" class="XYGraph (strict)"("Active Plot"=0, "Plot.YScaleIdx"=0, "Active Plot"=1, "Plot.YScaleIdx"=0) -> ()  [unwired: 2 in, 2 out]
              n155 = local write "LKG Path"(w85) -> ()
              n156 = local write "TRF Path"(w128) -> ()
            }
          }
        }
        frame #3 {
          n157 = local write "Status Indicator"(FALSE) -> ()
        }
        frame #4 {
          # "This frame creates the countdown timer for the wait inbetween the\nTransfer and Transport (if both selected)."
          n158 = disable-structure shown="Disabled" {
            frame Disabled {
              n159 = node-c288(1) -> (w225:T10)  [unwired: 1 in]
              n160 = timed-loop {
                timing: w225 -> [_]
                timing-out: [_] -> w224
                i -> [w236]
                stop <- w237 stop-if-true
                n161 = node-c288() -> ()  [unwired: 1 in, 1 out]
                n162 = local read "Wait Cluster"() -> (w229:T3)
                n163 = Unbundle By Name(w229) -> ("Wait Time (s)"=w227:dbl)
                n164 = Multiply(x=w236, y=0.001) -> (x*y=w234:dbl)
                n165 = local read "TRF Cluster"() -> (w230:T8)
                n166 = local read "TSP Cluster"() -> (w231:T9)
                n167 = Unbundle By Name(w231) -> ("Transport"=w232:bool)
                n168 = Unbundle By Name(w230) -> ("Transfer 2"=w233:bool)
                n169 = And(x=w233, y=w232) -> (x .and. y?=w241:bool)
                n170 = Select(t="Waiting...", s=w241, f="Ready") -> (s? t:f=w243:string)
                n171 = property on="Status Indicator" class="Bool (strict)"("BoolText.Text"=w243) -> ()  [unwired: 2 in, 2 out]
                n172 = Select(t=w227, s=w241, f=0) -> (s? t:f=w239:dbl)
                n173 = Subtract(x=w239, y=w234) -> (x-y=w228:dbl)
                n174 = Less Or Equal?(x=w228, y=0) -> (x <= y?=w237:bool)
                n175 = Bundle("Wait Time (s)"=w227, w228) -> (w226:cluster{"Wait Time (s)":dbl, dbl})  [unwired: 1 in]
                n176 = local write "Wait Cluster"(w226) -> ()
                n177 = node-c288() -> ()  [unwired: 1 in, 1 out]
              }
              n178 = node-c288(w224) -> ()  [unwired: 1 out]
            }
            frame Enabled {
            }
          }
        }
        frame #5 {
          n179 = local read "TSP Cluster"() -> (w252:T9)
          n180 = Unbundle By Name(w252) -> ("Transport"=w251:bool)
          n181 = case shown="True" w251 {
            frame False {
            }
            frame True {
              w285 = "XXX"
              w289 = "XXX"
              # "This frame takes the measurement settings and sends them to the Transport subVI for execution (if the \"Transport\" checkbox is selected on the front panel).\n\nThe data is saved to the folder specified by the user on the front panel with the file name generated by the sample properties.  If the file name already exists, the data is appended to the end of the file.\n\nThe Indicator LED on the front panel should display \"Measuring Transport\"."
              n182 = local read "Compliance Cluster"() -> (w264:T4)
              n183 = local read "TSP Cluster"() -> (w276:T9)
              n184 = local read "Gate Current Cluster"() -> (w254:T1)
              n185 = Unbundle By Name(w264) -> ("Var1 sweep settings 2"=w263:T13, "Var2 step settings 2"=w262:T14)
              n186 = local read "TSP Cluster"() -> (w269:T9)
              n187 = local read "VISA resource name"() -> (w266:refnum<visa-resource-name>)
              n188 = local read "TSP Cluster"() -> (w267:T9)
              n189 = Unbundle By Name(w267) -> ("Start"=w272:dbl, "Total Points"=w271:u16, "Step"=w270:dbl)
              n190 = Unbundle By Name(w276) -> ("Start 2"=w275:dbl, "Stop 3"=w274:dbl, "Step 2"=w273:dbl)
              n191 = Unbundle By Name(w269) -> ("Integration Time"=w268:u32)
              n192 = Unbundle By Name(w254) -> ("Gate Current (TSP)"=w253:T15)
              n193 = Unbundle(w263) -> ("sweep spacing (linear: 0)"=w312:u16, "sweep mode"=w311:bool, "compliance (V)"=w310:dbl, "compliance (A)"=w309:dbl)
              n194 = Bundle("Start 2"=w275, "Stop 3"=w274, "Step 2"=w273, "sweep spacing (linear: 0)"=w312, "sweep mode"=w311, "compliance (V)"=w310, "compliance (A)"=w309) -> (w308:T21)  [unwired: 1 in]
              n195 = Unbundle(w262) -> ("compliance (A)"=w307:dbl, "compliance (V)"=w306:dbl)
              n196 = local read "Saved Folder:"() -> (w265:path)
              n197 = Bundle("compliance (A)"=w307, "compliance (V)"=w306, "Start"=w272, "Total Points"=w271, "Step"=w270) -> (w305:T22)  [unwired: 1 in]
              n198 = local read "Sample Properties:"() -> (w301:T7)
              n199 = local write "Status Indicator"(TRUE) -> ()
              n200 = Build Path(base path=w265, name or relative path="TSP") -> (appended path=w278:path)
              n201 = Unbundle(w301) -> ("Index (#)"=w300:string, "Index (ABC)"=w299:string, "Length"=w290:string, "Width"=w286:string, "T (K)"=w260:dbl)  [unwired: 8 out]
              n202 = Equal?(x=w289, y=w290) -> (x = y?=w291:bool)
              n203 = property on="Status Indicator" class="Bool (strict)"("BoolText.Text"="Measuring\nTransport") -> ()  [unwired: 2 in, 2 out]
              n204 = Concatenate Strings(w300, w299) -> (w298:string)
              n205 = Equal?(x=w285, y=w286) -> (x = y?=w294:bool)
              n206 = local read "Graph Cluster"() -> (w258:T5)
              n207 = Decimal String To Number(string=w290) -> (number=w293:i32)  [unwired: 2 in, 1 out]
              n208 = Decimal String To Number(string=w286) -> (number=w292:i32)  [unwired: 2 in, 1 out]
              n209 = call <vilib>:"Check if File or Folder Exists.vi"("path"=w278) -> ("file or folder exists?"=w280:bool, "dup path"=w279:path)  [unwired: 8 in, 1 out]
              n210 = case shown="False" w280 {
                tunnel: w279 -> [w314 w315]
                tunnel: [w313 w315] -> w277
                frame False {
                  n211 = Create Folder(path (use dialog)=w314) -> (created path=w313:path)  [unwired: 2 in, 2 out]
                }
                frame True {
                }
              }
              n212 = Number To Decimal String(number=w293) -> (decimal integer string=w288:string)  [unwired: 1 in]
              n213 = Select(t=w289, s=w291, f=w288) -> (s? t:f=w287:string)
              n214 = Number To Decimal String(number=w292) -> (decimal integer string=w284:string)  [unwired: 1 in]
              n215 = Select(t=w285, s=w294, f=w284) -> (s? t:f=w283:string)
              n216 = call "Build Text2"("T"=w260, "Index"=w298, "Length"=w287, "Width"=w283) -> ("Result"=w282:string)  [unwired: 10 in, 1 out]
              n217 = Build Path(base path=w277, name or relative path=w282) -> (appended path=w295:path)
              n218 = call <vilib>:"Check if File or Folder Exists.vi"("path"=w295) -> ("file or folder exists?"=w297:bool, "dup path"=w296:path)  [unwired: 8 in, 1 out]
              n219 = case shown="True" w297 {
                tunnel: w296 -> [w316 w318]
                tunnel: [w316 w317] -> w261
                frame False {
                }
                frame True {
                  n220 = while {
                    tunnel: w318 -> [w320]
                    tunnel: [w319] -> w317
                    i -> [w322]
                    stop <- w323 stop-if-true
                    n221 = Path To String(path=w320) -> (string=w329:string)
                    n222 = Increment(x=w322) -> (x+1=w321:i32)
                    n223 = Number To Decimal String(number=w321) -> (decimal integer string=w327:string)  [unwired: 1 in]
                    n224 = Concatenate Strings(w329, "_", w327) -> (w326:string)
                    n225 = String To Path(string=w326) -> (path=w325:path)
                    n226 = call <vilib>:"Check if File or Folder Exists.vi"("path"=w325) -> ("file or folder exists?"=w324:bool, "dup path"=w319:path)  [unwired: 8 in, 1 out]
                    n227 = Not(x=w324) -> (.not. x?=w323:bool)
                  }
                }
              }
              n228 = call "transport char run_subvi_2013_09_11_JWa.vi"("VISA session"=w266, "Y2 axis settings"=w253, "Var1 sweep settings"=w308, "Var2 step settings"=w305, "integration time"=w268, "Path"=w261, "Sample Properties:"=w301) -> ("Graph Cluster"=w259:T23, "error?"=w304:errorcluster)  [unwired: 6 in, 1 out]
              n229 = local write "error out"(w304) -> ()
              n230 = Unbundle By Name(w259) -> ("Transport"=w256:cluster{dbl[], dbl[]}[], "Gate Current"=w255:cluster{dbl[], dbl[]}[])
              n231 = local write "TSP Path"(w261) -> ()
              n232 = Bundle By Name(cluster=w258, "Transport"=w256, "TSP Gate Current"=w255) -> (w257:T5)
              n233 = local write "Graph Cluster"(w257) -> ()
            }
          }
        }
        frame #6 {
          n234 = local write "Status Indicator"(FALSE) -> ()
          n235 = property on="Status Indicator" class="Bool (strict)"("BoolText.Text"="Ready") -> ()  [unwired: 2 in, 2 out]
        }
        frame #7 {
          n236 = disable-structure shown="Disabled" {
            disable-tunnel: w333 -> [w335 _]
            disable-tunnel: w332 -> [w334 _]
            frame Disabled {
              n237 = node-c288(100) -> (w340:T10)  [unwired: 3 in]
              n238 = timed-loop {
                timing: w340 -> [_]
                timing-out: [_] -> w339
                tunnel: w335 -> [w351]
                tunnel: w334 -> [w350]
                tunnel: ["Stop \nCountdown"] -> _
                i -> [w356]
                stop <- w346 stop-if-true
                n239 = node-c288() -> ()  [unwired: 1 in, 1 out]
                n240 = local read "TRF Cluster"() -> (w345:T8)
                n241 = Unbundle By Name(w345) -> ("Loop Wait"=w343:dbl)
                n242 = Multiply(x=0.1, y=w356) -> (x*y=w354:dbl)
                n243 = Equal?(x=w350, y=w351) -> (x = y?=w352:bool)
                n244 = Select(t=0, s=w352, f=w343) -> (s? t:f=w348:dbl)
                n245 = Subtract(x=w348, y=w354) -> (x-y=w342:dbl)
                n246 = Less Or Equal To 0?(x=w342) -> (x <= 0?=w347:bool)
                n247 = Or(x=w347, y="Stop \nCountdown") -> (x .or. y?=w346:bool)
                n248 = Bundle("Loop Wait"=w343, w342) -> (w344:cluster{"Loop Wait":dbl, dbl})  [unwired: 1 in]
                n249 = property on="Status Indicator" class="Bool (strict)"("BoolText.Text"="Waiting...") -> ()  [unwired: 2 in, 2 out]
                n250 = local write "Wait Cluster"(w344) -> ()
                n251 = node-c288() -> ()  [unwired: 1 in, 1 out]
              }
              n252 = node-c288(w339) -> (w336:errorcluster)
              n253 = property on="Status Indicator" class="Bool (strict)"(error in=w336, "BoolText.Text"="Ready") -> ()  [unwired: 1 in, 2 out]
            }
            frame Enabled {
            }
          }
        }
      }
      n254 = local write "VISA resource name out"(w9) -> ()
    }
  }
